vi "Increase command Date.vi"(11 "Cluster 2":T1) -> (3 "Cluster 2":T1)   [LabVIEW 2020, in "CSM-ScheduledCmdWindow.lvlib"]
uses:
  CSM-ScheduledCmdWindow.lvlib
  Command Timer Item.ctl
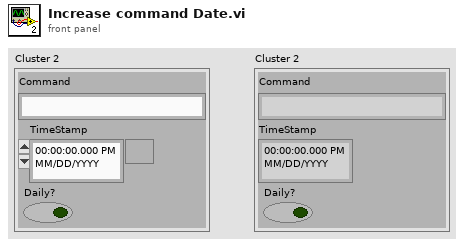
[diagram p1: front panel]
types:
  T1 = typedef "CSM-ScheduledCmdWindow.lvlib/Command Timer Item.ctl" = cluster{"Command":string, "TimeStamp":timestamp, "Daily?":bool}
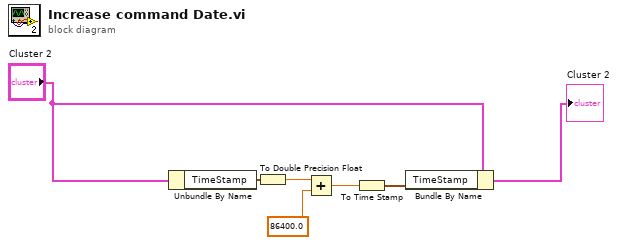
[diagram p0: block diagram]
diagram:
  n1 = Unbundle By Name("Cluster 2") -> ("TimeStamp"=w7:timestamp)
  n2 = To Double Precision Float(number=w7) -> (double precision float=w6:dbl)
  n3 = Add(x=w6, y=86400.0) -> (x+y=w3:dbl)
  n4 = To Time Stamp(1:w3) -> (0:w2:timestamp)
  n5 = Bundle By Name(cluster="Cluster 2", "TimeStamp"=w2) -> (→"Cluster 2":T1)
